vi "Linear sweep (linspace).vi"(1 "Stop frequency":dbl, 2 "Start frequency":dbl, 3 "Number of points":i32=2 min=2) -> (0 "linspace":dbl[](array[numeric]))   [LabVIEW 2021]
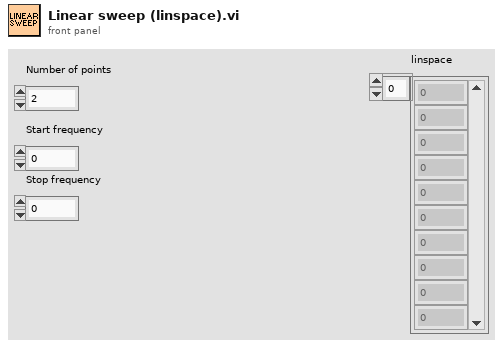
[diagram p1: front panel]
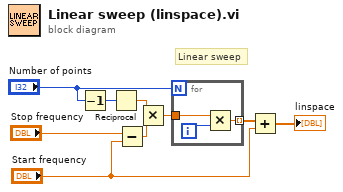
[diagram p0: block diagram]
diagram:
  # "Linear sweep"
  n1 = Decrement(x="Number of points") -> (x-1=w1:i32)
  n2 = Reciprocal(x=w1) -> (1/x=w6:dbl)
  n3 = Subtract(x="Stop frequency", y="Start frequency") -> (x-y=w8:dbl)
  n4 = Multiply(x=w6, y=w8) -> (x*y=w5:dbl)
  n5 = for {
    N: "Number of points" -> [_]
    tunnel: w5 -> [w12]
    tunnel: [w11] -> w4 mode=indexing
    i -> [w10]
    n6 = Multiply(x=w12, y=w10) -> (x*y=w11:dbl)
  }
  n7 = Add(x=w4, y="Start frequency") -> (x+y=→"linspace":dbl[])
